vi "Request UI Display.vi"(6 "wait for reply (T)":bool=TRUE, 8 "error in (no error)":errorcluster, 10 "Scenario":T1) -> (0 "error out":errorcluster, 3 "Accept?":bool)   [LabVIEW 2022 SP3, in "Dummy.lvlib"]
doc: "Requests the module to display its UI as specified in <b>Scenario</b>:\n\"managed\" => in the UI Manager's subpanel\n\"stand-alone\" => as a separate window\n____\nHAMPEL SOFTWARE ENGINEERING v2.6.0 (2023-12-19 10:54)"
uses:
  Dummy.lvlib
  Libraries/hse-libraries/Source/hse-dqmh/Controls/Module Display Scenarios.ctl
  Request UI Display Argument--cluster.ctl
  Request UI Display (Reply Payload)--cluster.ctl
  Libraries/hse-libraries/Source/hse-dqmh/hse-dqmh.lvlib
panel:
  out "timed out?":bool
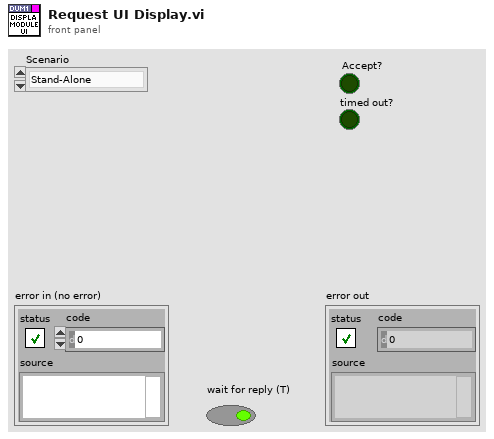
[diagram p1: front panel]
types:
  T1 = typedef "hse-dqmh.lvlib/Module Display Scenarios.ctl" = enum16{"Stand-Alone", "Managed"}
  T2 = typedef "Dummy.lvlib/Request UI Display Argument--cluster.ctl" = cluster{"Scenarios":T1, "Wait Notifier":refnum<notifier>, "wait for reply":bool}
  T3 = typedef "Dummy.lvlib/Request Events--cluster.ctl" = cluster{"Stop Module":refnum<user-event>, "Show Panel":refnum<user-event>, "Hide Panel":refnum<user-event>, "Get Module Execution Status":refnum<user-event>, "Show Diagram":refnum<user-event>, "Configure":refnum<user-event>, "Prepare":refnum<user-event>, "Register for UI Login":refnum<user-event>, "Request UI Display":refnum<user-event>}
  T4 = typedef "Dummy.lvlib/Request UI Display (Reply Payload)--cluster.ctl" = cluster{"Accept?":bool, "Error":errorcluster}
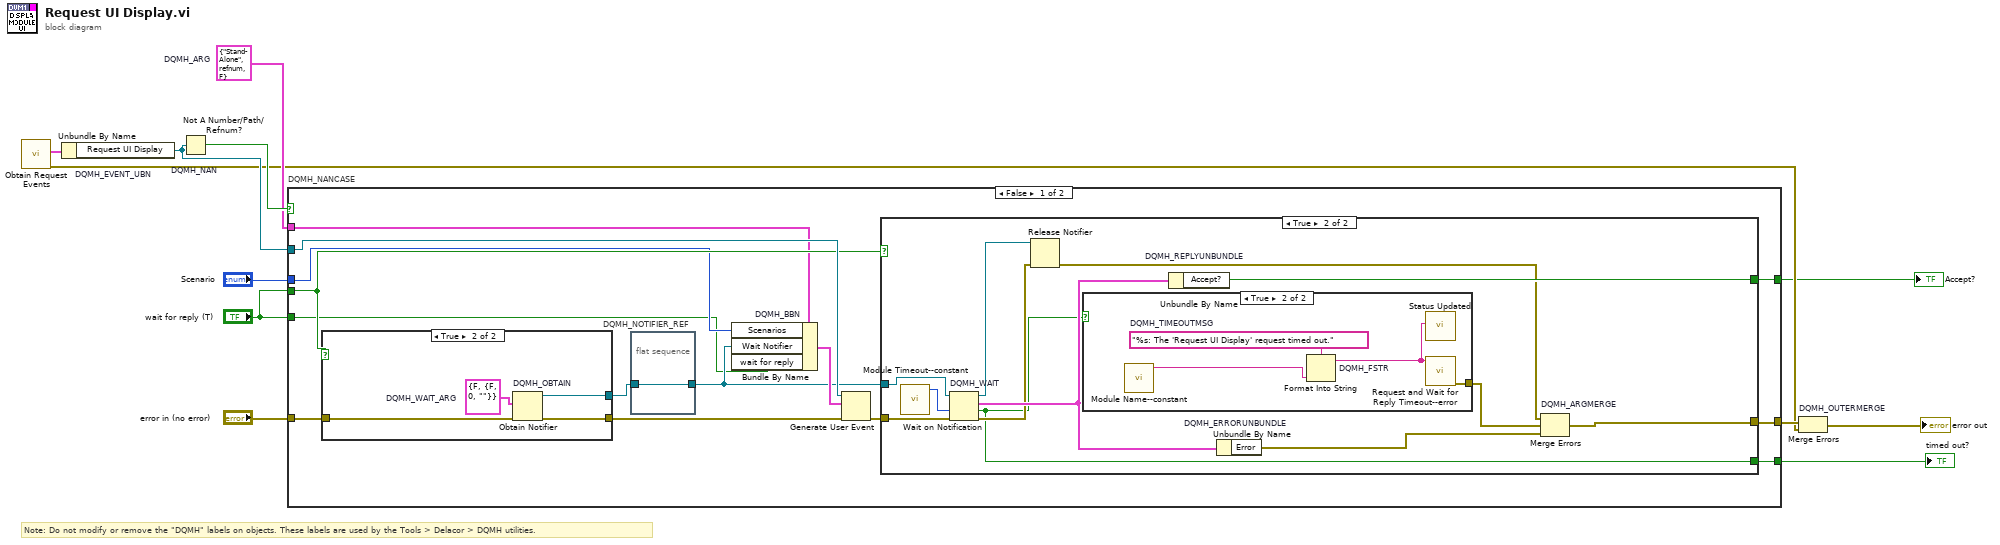
[diagram p0: block diagram]
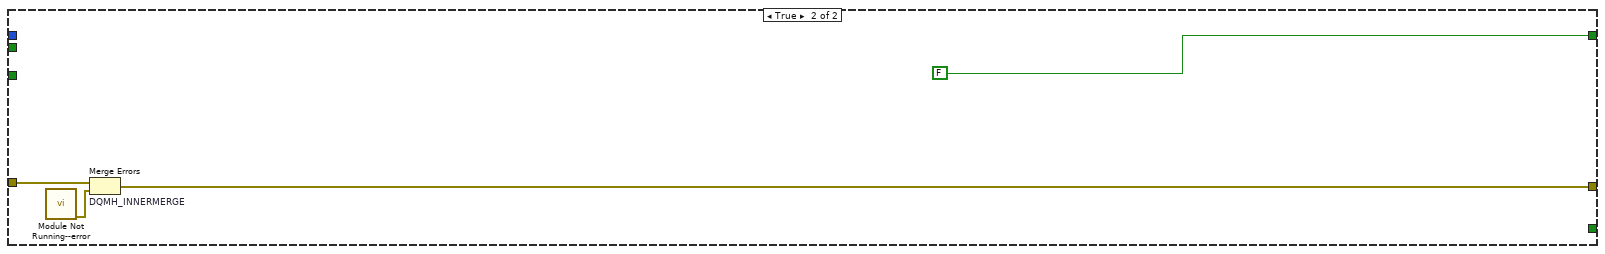
[diagram p5: hidden frame]
diagram:
  w7 = T2 {"Scenarios"=enum."Stand-Alone", "Wait Notifier"=refnum, "wait for reply"=FALSE}  # DQMH_ARG
  # "Note: Do not modify or remove the \"DQMH\" labels on objects. These labels are used by the Tools > Delacor > DQMH utilities."
  n1 = call "Obtain Request Events.vi"() -> ("error out"=w4:errorcluster, "Dummy Request Events"=w3:T3)  [unwired: 10 in]
  n2 = Unbundle By Name "DQMH_EVENT_UBN"(w3) -> ("Request UI Display"=w8:refnum<user-event>)
  n3 = Not A Number/Path/Refnum? "DQMH_NAN"(number/path/refnum=w8) -> (NaN/Path/Refnum?=w9:bool)
  n4 = case "DQMH_NANCASE" shown="False" w9 {
    tunnel: "error in (no error)" -> [w26 w54]
    tunnel: w8 -> [w24 _]
    tunnel: [w22 w53] -> w10
    tunnel: "wait for reply (T)" -> [w20 _]
    tunnel: w7 -> [w17 _]
    tunnel: "Scenario" -> [w16 _]
    tunnel: "wait for reply (T)" -> [w15 _]
    tunnel: [w14 FALSE] -> w2
    tunnel: [w13 _] -> w1
    frame False {
      n5 = case shown="True" w20 {
        tunnel: w26 -> [w46 w50]
        tunnel: [w46 w49] -> w23
        tunnel: [_ w47] -> w19
        frame False {
        }
        frame True {
          w48 = T4 {"Accept?"=FALSE, "Error"={"status"=FALSE, "code"=0, "source"=""}}  # DQMH_WAIT_ARG
          n6 = Obtain Notifier "DQMH_OBTAIN"(notification data type=w48, error in (no error)=w50) -> (notifier out=w47:refnum<notifier>, error out=w49:errorcluster)  [unwired: 2 in, 1 out]
        }
      }
      n7 = flat-sequence "DQMH_NOTIFIER_REF" {
        tunnel: w19 -> [w27]
        tunnel: [w27] -> w18
        frame #0 {
        }
      }
      n8 = Bundle By Name "DQMH_BBN"(cluster=w17, "Scenarios"=w16, "Wait Notifier"=w18, "wait for reply"=w15) -> (w21:T2)
      n9 = Generate User Event(user event=w24, event data cluster=w21, error in=w23) -> (error out=w25:errorcluster)  [unwired: 1 in, 1 out]
      n10 = case shown="True" w20 {
        tunnel: w25 -> [w29 w41]
        tunnel: w18 -> [_ w40]
        tunnel: [w29 w38] -> w22
        tunnel: [w28 w34] -> w14
        tunnel: [_ w30] -> w13
        frame False {
          w28 = FALSE  # Accept?
        }
        frame True {
          n11 = call "Module Timeout--constant.vi"() -> ("Module Timeout"=w36:i32)  [unwired: 11 in]
          n12 = Wait on Notification "DQMH_WAIT"(notifier=w40, timeout in ms (-1)=w36, error in (no error)=w41) -> (notifier out=w39:refnum<notifier>, notification=w35:T4, timed out?=w30:bool, error out=w33:errorcluster)  [unwired: 1 in]
          n13 = Release Notifier(notifier=w39, error in (no error)=w33) -> (error out=w31:errorcluster)  [unwired: 1 in, 2 out]
          n14 = case shown="True" w30 {
            tunnel: [_ w43] -> w32
            frame False {
            }
            frame True {
              w45 = "%s: The 'Request UI Display' request timed out."  # DQMH_TIMEOUTMSG
              n15 = call "Module Name--constant.vi"() -> ("Module Name"=w42:string)  [unwired: 11 in]
              n16 = Format Into String "DQMH_FSTR"(format string=w45, w42) -> (resulting string=w44:string)  [unwired: 2 in, 1 out]
              n17 = call "Status Updated.vi"("Status"=w44) -> ()  [unwired: 10 in, 1 out]
              n18 = call "Request and Wait for Reply Timeout--error.vi"("Error Message"=w44) -> ("error out"=w43:errorcluster)  [unwired: 10 in]
            }
          }
          n19 = Unbundle By Name "DQMH_REPLYUNBUNDLE"(w35) -> ("Accept?"=w34:bool)
          n20 = Unbundle By Name "DQMH_ERRORUNBUNDLE"(w35) -> ("Error"=w37:errorcluster)
          n21 = Merge Errors "DQMH_ARGMERGE"(w31, w32, w37) -> (w38:errorcluster)
        }
      }
    }
    frame True {
      n22 = call "Module Not Running--error.vi"() -> ("error out"=w52:errorcluster)  [unwired: 11 in]
      n23 = Merge Errors "DQMH_INNERMERGE"(w54, w52) -> (w53:errorcluster)
    }
  }
  "Accept?" <- w2
  "timed out?" <- w1
  n24 = Merge Errors "DQMH_OUTERMERGE"(w10, w4) -> (→"error out":errorcluster)
